vi "Create Client.vi"(8 "error in":errorcluster, 11 "cluster id":string) -> (0 "error out":errorcluster, 3 "grpc client id":T1)   [LabVIEW 2021, in "NI Discovery V1 Client.lvlib"]
uses:
  NI Discovery V1 Client.lvlib
  gRPC/Generated APIs/ni/measurementlink/discovery/v1/ni.measurementlink.discovery.v1.api.lvlib
  <vilib>/gRPC/LabVIEW gRPC Library/Shared/grpcId.ctl
  <vilib>/gRPC/LabVIEW gRPC Library/grpc-lvsupport-release.lvlib
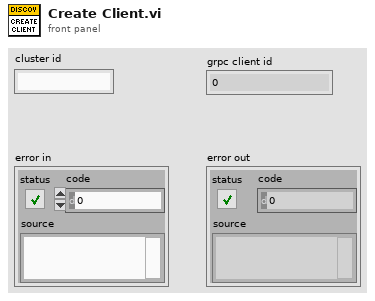
[diagram p1: front panel]
types:
  T1 = typedef "grpc-lvsupport-release.lvlib/grpcId.ctl" = u64
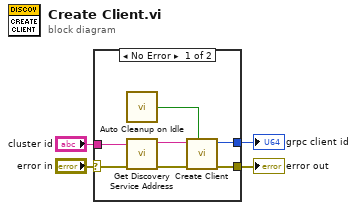
[diagram p0: block diagram]
diagram:
  n1 = case shown="No Error" "error in" {
    selector: "error in" -> [w9 w12]
    tunnel: [w11 _] -> w4
    tunnel: [w10 w12] -> w3
    tunnel: "cluster id" -> [w6 _]
    frame No Error {
      n2 = call "Auto Cleanup on Idle.vi"() -> ("auto cleanup"=w5:bool)  [unwired: 1 in]
      n3 = call "Get Discovery Service Address.vi"("error in"=w9, "cluster id (\"\")"=w6) -> ("error out"=w7:errorcluster, "address"=w8:string)  [unwired: 8 in]
      n4 = call "Create Client.vi"("auto cleanup"=w5, "error in"=w7, "address"=w8) -> ("error out"=w10:errorcluster, "gRPC ID Out"=w11:T1)  [unwired: 7 in]
    }
    frame Error {
    }
  }
  "grpc client id" <- w4
  "error out" <- w3
